vi "Find Workspace.vi"(8 "Error In":errorcluster, 10 "Control In":T2, 11 "Carrier Tray in":refnum<class "Assembly Tray.lvclass">) -> (0 "Error Out":errorcluster, 1 "Workspace":T1, 2 "Control Out":T2, 3 "Carrier Tray Out":refnum<class "Assembly Tray.lvclass">)   [LabVIEW 2019, in "Assembly Tray.lvclass"]
uses:
  Assembly Tray.lvclass
  C:/Users/HEP/Documents/Aerotech gantry/UCSB-Gantry-master-main/V5/Classes/Workspace/Fixture.lvclass
  Controller/Controllers.ctl
  Controller/I-O/I-O.lvclass
  Controller/Dispenser/Dispenser.lvclass
  C:/Program Files (x86)/Aerotech/A3200/LabVIEW/2010/Bin/Aerotech.A3200.dll
  Program Files (x86)/Aerotech/A3200/LabVIEW/2010/Bin/Aerotech.A3200.dll
  Workspace.ctl
  Fixture.lvclass/Fixture.ctl
  Assembly Tray.lvclass/Assembly Tray.ctl
  Read Fixture ID.vi
  Fixture.lvclass
  Controller/Controller.lvclass
panel:
  in  "output cluster 2":T1
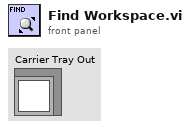
[diagram p1: front panel]
types:
  T1 = typedef "Fixture.lvclass/Workspace.ctl" = cluster{"XYZTheta":dbl[], "Workspace Valve":i32, "Workspace Sensor":i32}
  T2 = typedef "Controller.lvclass/Controllers.ctl" = cluster{"I-O.lvclass":refnum<class "I-O.lvclass">, "Dispenser.lvclass":refnum<class "Dispenser.lvclass">, "Gantry":refnum<k24>}
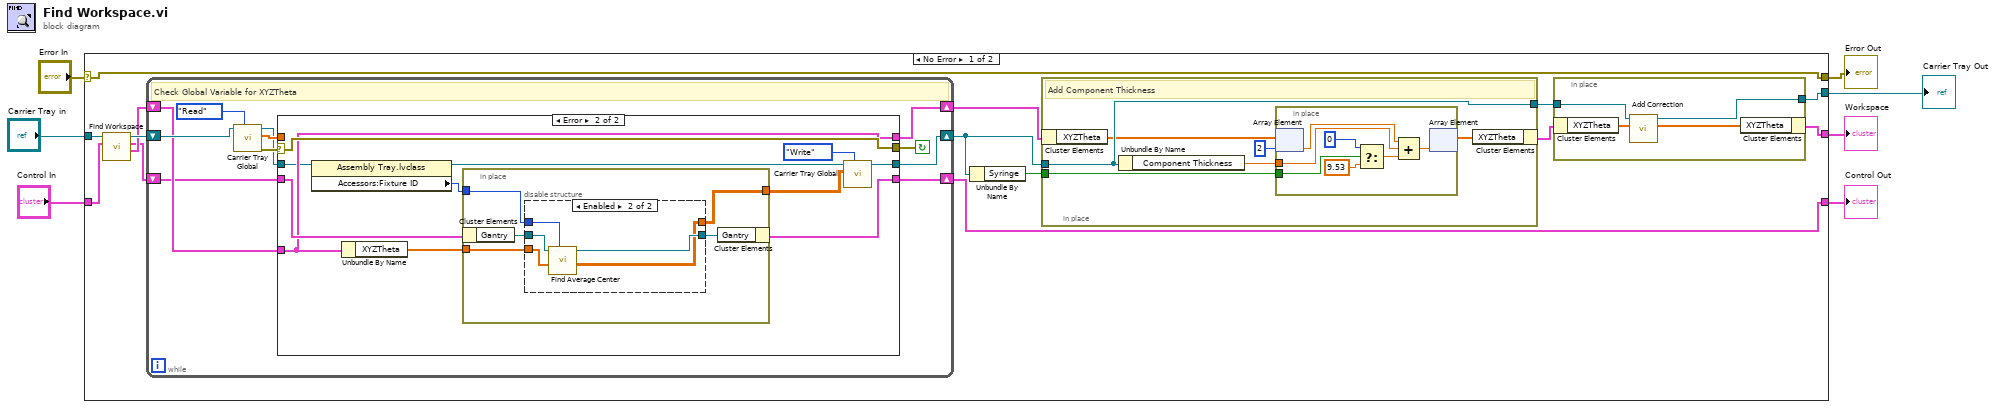
[diagram p0: block diagram]
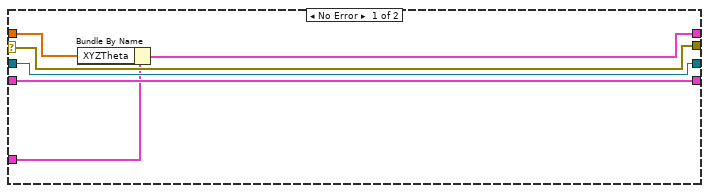
[diagram p2: hidden frame]
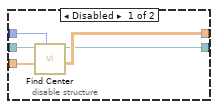
[diagram p3: hidden frame]
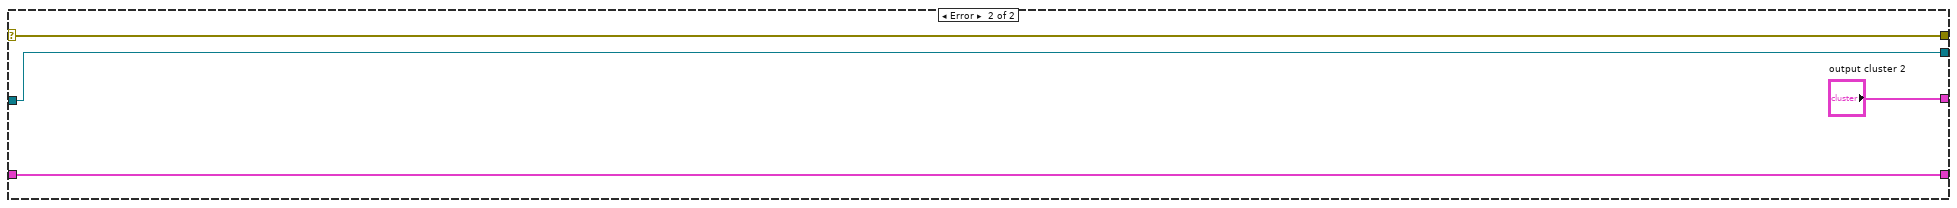
[diagram p4: hidden frame]
diagram:
  n1 = case shown="No Error" "Error In" {
    selector: "Error In" -> [w21 w84]
    tunnel: [w21 w84] -> w6
    tunnel: "Control In" -> [w20 w85]
    tunnel: [w16 w85] -> w4
    tunnel: "Carrier Tray in" -> [w19 w82]
    tunnel: [w17 "output cluster 2"] -> w2
    tunnel: [w18 w82] -> w1
    frame No Error {
      n2 = call-parent "Find Workspace.vi"("Control In"=w20, "Workspace In"=w19) -> (1:"Workspace Out"=w14:T1, "Control Out"=w13:T2, 3:"Workspace Out"=w15:refnum<class "Assembly Tray.lvclass">)  [unwired: 6 in, 1 out]
      n3 = while {
        shift-right: [w40] -> w12
        shift-left: w15 -> [w48]
        shift-right: [w42] -> w16
        shift-left: w13 -> [w43]
        shift-right: [w39] -> w11
        shift-left: w14 -> [w44]
        stop <- w46 continue-if-true
        # "Check Global Variable for XYZTheta"
        n4 = call "Carrier Tray Global.vi"("Action"=enum16{"Initialize", "Read", "Write"}."Read", "Carrier Tray.lvclass"=w48) -> ("error out"=w47:errorcluster, "XYZTheta out"=w45:dbl[], "Carrier Tray.lvclass 2"=w41:refnum<class "Assembly Tray.lvclass">)  [unwired: 7 in]
        n5 = case shown="Error" w47 {
          selector: w47 -> [w55 w66]
          tunnel: [w55 w66] -> w46
          tunnel: w45 -> [w52 _]
          tunnel: [w54 w61] -> w39
          tunnel: w44 -> [w50 w61]
          tunnel: w43 -> [w51 w65]
          tunnel: [w51 w64] -> w42
          tunnel: w41 -> [w53 w59]
          tunnel: [w53 w63] -> w40
          frame No Error {
            n6 = Bundle By Name(cluster=w50, "XYZTheta"=w52) -> (w54:T1)
          }
          frame Error {
            n7 = property class="Assembly Tray.lvclass"(reference=w59) -> (reference out=w58:refnum<class "Assembly Tray.lvclass">, "Accessors:Fixture ID"=w57:i32)  [unwired: 1 in, 1 out]
            n8 = Unbundle By Name(w61) -> ("XYZTheta"=w60:dbl[])
            n9 = in-place {
              in-place-border: [w71] -> w56
              in-place-border: w60 -> [w70]
              in-place-border: w57 -> [w69]
              n10 = in-place-cluster #1(w65) -> ("Gantry"=w68:refnum<k24>)
              n11 = disable-structure shown="Enabled" {
                disable-tunnel: [w76 w77] -> w71
                disable-tunnel: w70 -> [w72 w79]
                disable-tunnel: w69 -> [w75 w78]
                disable-tunnel: w68 -> [w74 w81]
                disable-tunnel: [w73 w80] -> w67
                frame Disabled {
                  n12 = call "Find Center.vi"("Tray Number"=w75, "XYZTheta"=w72, "Gantry In"=w74) -> ("XYZTheta Centers"=w76:dbl[][], "Gantry Out"=w73:refnum<k24>)  [unwired: 7 in]
                }
                frame Enabled {
                  n13 = call "Find Average Center.vi"("Tray Number"=w78, "XYZTheta"=w79, "Gantry In"=w81) -> ("XYZTheta Centers"=w77:dbl[][], "Gantry Out"=w80:refnum<k24>)  [unwired: 7 in]
                }
              }
              n14 = in-place-cluster #1("Gantry"=w67) -> (w64:T2)
            }
            n15 = call "Carrier Tray Global.vi"("Action"=enum16{"Initialize", "Read", "Write"}."Write", "XYZTheta in"=w56, "Carrier Tray.lvclass"=w58) -> ("Carrier Tray.lvclass 2"=w63:refnum<class "Assembly Tray.lvclass">)  [unwired: 6 in, 2 out]
          }
        }
      }
      n16 = Unbundle By Name(w12) -> ("Syringe"=w10:bool)
      n17 = in-place {
        in-place-border: w12 -> [w24]
        in-place-border: [w24] -> w9
        in-place-border: w10 -> [w23]
        # "Add Component Thickness"
        n18 = in-place-cluster #2(w11) -> ("XYZTheta"=w22:dbl[])
        n19 = Unbundle By Name(w24) -> ("Component Thickness"=w25:dbl)
        n20 = in-place {
          in-place-border: w25 -> [w33]
          in-place-border: w23 -> [w31]
          n21 = in-place-array #3(w22, 2) -> (w34:dbl)
          n22 = Select(t=0, s=w31, f=9.53) -> (s? t:f=w28:dbl)
          n23 = Compound Arithmetic op=ADD(w34, w33, w28) -> (w32:dbl)
          n24 = in-place-array #3(w32) -> (w26:dbl[])  [unwired: 1 out]
        }
        n25 = in-place-cluster #2("XYZTheta"=w26) -> (w8:T1)
      }
      n26 = in-place {
        in-place-border: [w38] -> w18
        in-place-border: w9 -> [w37]
        n27 = in-place-cluster #4(w8) -> ("XYZTheta"=w36:dbl[])
        n28 = call "Add Correction.vi"("XYZTheta"=w36, "Carrier Tray in"=w37) -> ("XYZTheta Out"=w35:dbl[], "Carrier Tray out"=w38:refnum<class "Assembly Tray.lvclass">)  [unwired: 7 in, 1 out]
        n29 = in-place-cluster #4("XYZTheta"=w35) -> (w17:T1)
      }
    }
    frame Error {
    }
  }
  "Error Out" <- w6
  "Control Out" <- w4
  "Workspace" <- w2
  "Carrier Tray Out" <- w1
